vi "Hold.vi"(6 "Axis":T1, 8 "error in (no error)":errorcluster, 11 "Instrument.VRM in":refnum<class "Instrument.OxfordVRM.lvclass">) -> (0 "error out":errorcluster, 2 "Response":string, 3 "Instrument.VRM out":refnum<class "Instrument.OxfordVRM.lvclass">)   [LabVIEW 2016, in "Instrument.OxfordVRM.lvclass"]
uses:
  Instrument.OxfordVRM.lvclass
  <userlib>/LevyLab/Levylab Instruments/Instrument Types/Cryostat/Typedefs/Magnet Axis--Enum.ctl
  <instrlib>/Mercury iXX/Public/Libraries/Magnet/Controls/PSU Actions.ctl
  Typedefs/Instrument.Oxford1820.Commands-enum.ctl
  Typedefs/VRM Action-Axis--Cluster.ctl
  <userlib>/LevyLab/Levylab Instruments/Instrument Types/Cryostat/Typedefs/VRM Magnet Axis--Enum.ctl
  <instrlib>/Mercury iXX/Public/Libraries/Magnet.lvlib
  <userlib>/LevyLab/Levylab Instruments/Instrument Types/Cryostat/Instrument.Cryostat.lvclass
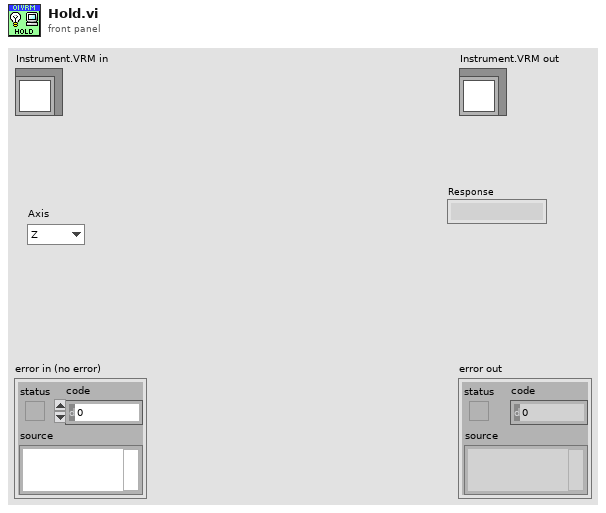
[diagram p1: front panel]
types:
  T1 = typedef "Instrument.Cryostat.lvclass/Magnet Axis--Enum.ctl" = enum16{"Z", "X", "Y"}
  T2 = typedef "Instrument.OxfordVRM.lvclass/VRM Action-Axis--Cluster.ctl" = cluster{"PSU Act Stat":T3, "Axis":T4}
  T3 = typedef "Mercury iXX.lvlib/Magnet.lvlib/PSU Actions.ctl" = string
  T4 = typedef "Instrument.OxfordVRM.lvclass/VRM Magnet Axis--Enum.ctl" = enum16{"Z", "X", "Y", "ALL"}
  T5 = typedef "Instrument.OxfordVRM.lvclass/Instrument.Oxford1820.Commands-enum.ctl" = enum16{"setAction", "setTarget", "setMagnetField", "getStatus", "getTarget", "getMagnetField"}
  T6 = cluster{"Holding":bool, "Ramp to Setpoint":bool, "Ramp to Zero":bool, "Clamp":bool}
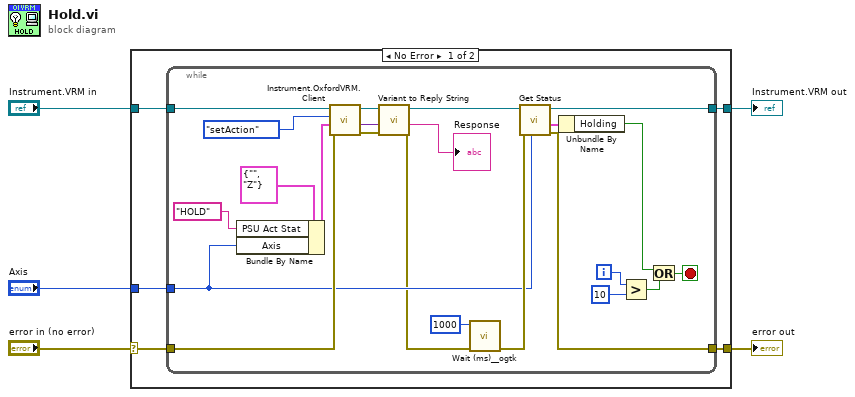
[diagram p0: block diagram]
diagram:
  n1 = case shown="No Error" "error in (no error)" {
    selector: "error in (no error)" -> [w9 w35]
    tunnel: [w7 w35] -> w4
    tunnel: [w8 w34] -> w2
    tunnel: "Instrument.VRM in" -> [w10 w34]
    tunnel: "Axis" -> [w6 _]
    frame No Error {
      n2 = while {
        tunnel: w6 -> [w12]
        tunnel: w10 -> [w28]
        tunnel: [w27] -> w8
        tunnel: w9 -> [w33]
        tunnel: [w32] -> w7
        i -> [w22]
        stop <- w24 stop-if-true
        n3 = Bundle By Name(cluster=T2 {"PSU Act Stat"="", "Axis"=enum."Z"}, "PSU Act Stat"=T3 "HOLD", "Axis"=w12) -> (w14:T2)
        n4 = call "Instrument.OxfordVRM.Client.vi"("error in (no error)"=w33, "Data"=w14, "Commands"=Instrument.Oxford1820.Commands-enum."setAction", "Instrument.VRM in"=w28) -> ("error out"=w17:errorcluster, "Data out"=w19:variant, "Instrument.VRM out"=w21:refnum<class "Instrument.OxfordVRM.lvclass">)  [unwired: 5 in]
        n5 = call "Variant to Reply String.vi"("error in (no error)"=w17, "Data"=w19, "Instrument.VRM in"=w21) -> ("error out"=w11:errorcluster, "Reply"=→"Response":string, "Instrument.VRM out"=w20:refnum<class "Instrument.OxfordVRM.lvclass">)  [unwired: 6 in]
        n6 = call <userlib>:"Wait (ms)__ogtk.vi"("error in (no error)"=w11, "milliseconds to wait"=u32 1000) -> ("error out"=w31:errorcluster)  [unwired: 8 in, 1 out]
        n7 = call "Get Status.vi"("Axis"=w12, "error in (no error)"=w31, "Instrument.VRM in"=w20) -> ("error out"=w32:errorcluster, "Status"=w29:T6, "Instrument.VRM out"=w27:refnum<class "Instrument.OxfordVRM.lvclass">)  [unwired: 5 in, 1 out]
        n8 = Unbundle By Name(w29) -> ("Holding"=w23:bool)
        n9 = Greater?(x=w22, y=10) -> (0:w25:bool)
        n10 = Or(x=w23, y=w25) -> (x .or. y?=w24:bool)
      }
    }
    frame Error {
    }
  }
  "error out" <- w4
  "Instrument.VRM out" <- w2
